vi "findNodesFromPath.vi"(8 "error in (no error)":errorcluster, 10 "searchInElement":string="/device_settings/analog_output name=\"Ao32\"", 11 "xmlNode in":refnum<class "xmlNode.lvclass">) -> (0 "error out":errorcluster, 1 "rest of xml":string, 2 "xmlNode":refnum<class "xmlNode.lvclass">, 3 "xmlNode out":refnum<class "xmlNode.lvclass">, 5 "xml before":string)   [LabVIEW 2011, in "Tools.lvlib" / "xml.lvlib" / "xmlNode.lvclass"]
uses:
  xmlNode.lvclass
  XmlParser.lvclass
panel:
  out "xml":string
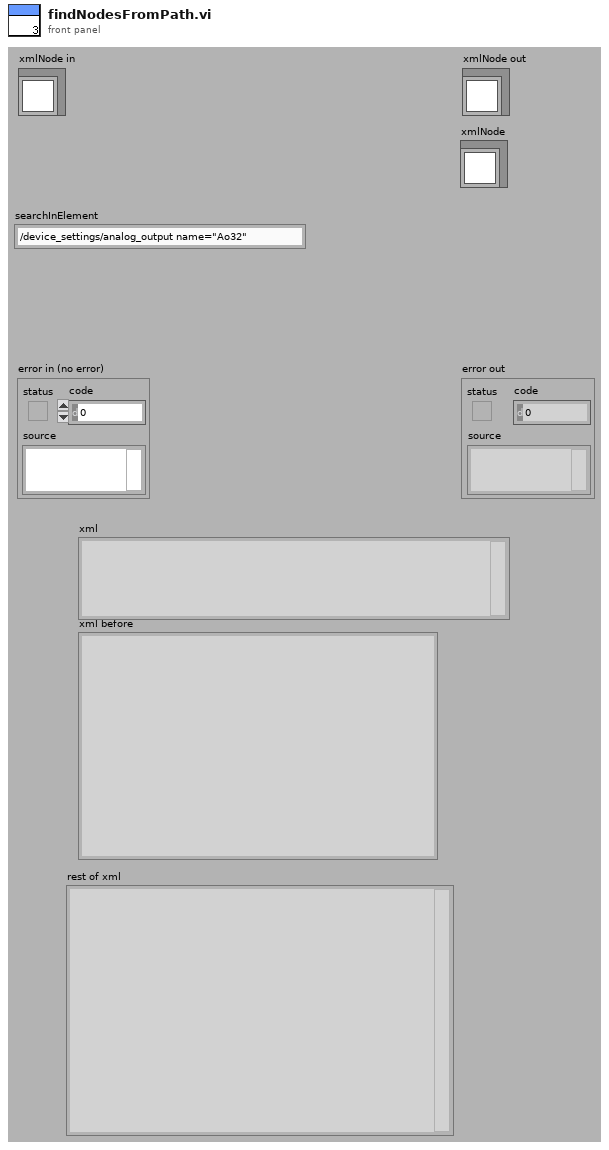
[diagram p1: front panel]
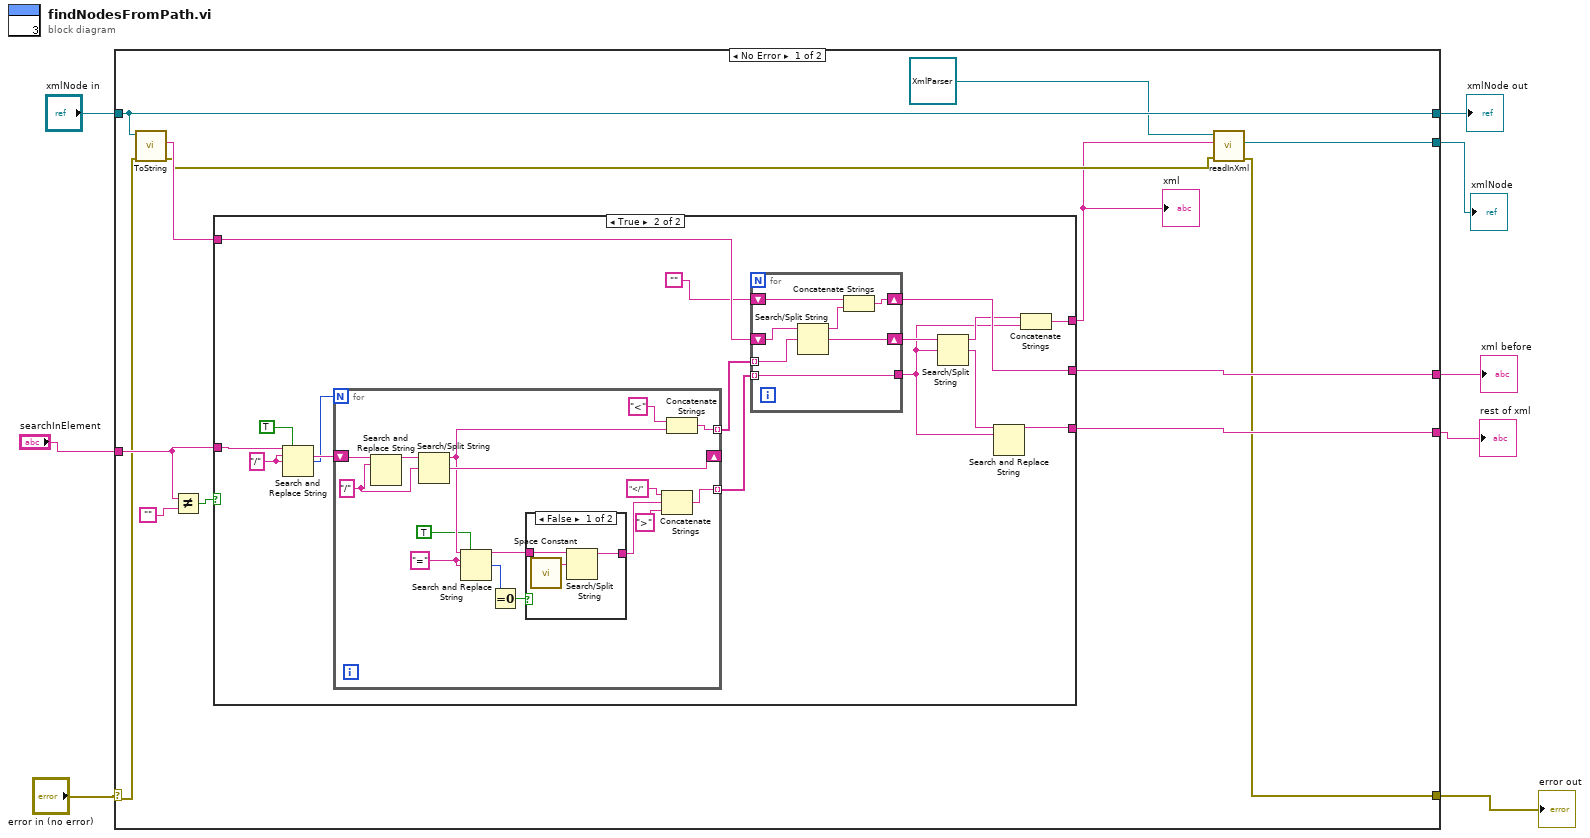
[diagram p0: block diagram]
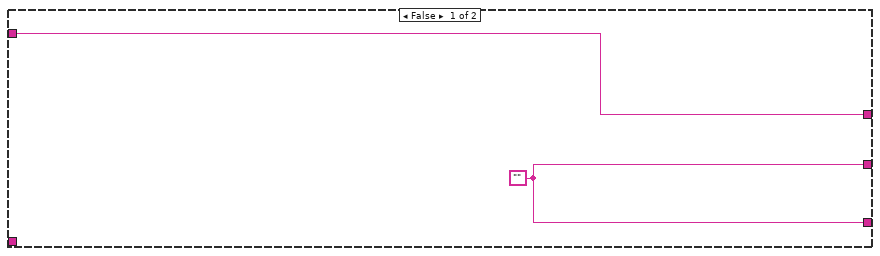
[diagram p2: hidden frame]
diagram:
  n1 = case shown="No Error" "error in (no error)" {
    selector: "error in (no error)" -> [w12 w68]
    tunnel: [w10 w68] -> w7
    tunnel: [w18 w67] -> w5
    tunnel: "xmlNode in" -> [w18 w67]
    tunnel: "searchInElement" -> [w19 _]
    tunnel: [w16 _] -> w2
    tunnel: [w15 _] -> w1
    tunnel: [w11 _] -> w3
    frame No Error {
      n2 = call-dynamic "ToString.vi"("error in (no error)"=w12, "xmlNode in"=w18) -> ("error out"=w13:errorcluster, "xml"=w17:string)  [unwired: 7 in, 1 out]
      n3 = Not Equal?(x=w19, y="") -> (x != y?=w20:bool)
      n4 = case shown="True" w20 {
        tunnel: [w22 w34] -> w9
        tunnel: w19 -> [_ w35]
        tunnel: [w23 w24] -> w15
        tunnel: [w23 w30] -> w16
        tunnel: w17 -> [w22 w32]
        frame False {
          w23 = ""
        }
        frame True {
          w37 = "/"
          n5 = Search and Replace String(replace all?=TRUE, input string=w35, search string=w37, replace string=w37) -> (result string=w39:string, number of replacements=w38:i32)  [unwired: 4 in, 2 out]
          n6 = for {
            N: w38 -> [_]
            tunnel: [w56] -> w33 mode=indexing
            tunnel: [w55] -> w27 mode=indexing
            shift-right: [w54] -> _
            shift-left: w39 -> [w62]
            w52 = "="
            w61 = "/"
            n7 = Search and Replace String(input string=w62, search string=w61) -> (result string=w60:string)  [unwired: 6 in, 3 out]
            n8 = Search/Split String(string=w60, search string/char (-)=w61) -> (substring before match=w53:string, match + rest of string=w54:string)  [unwired: 1 in, 1 out]
            n9 = Search and Replace String(replace all?=TRUE, input string=w53, search string=w52, replace string=w52) -> (result string=w49:string, number of replacements=w51:i32)  [unwired: 4 in, 2 out]
            n10 = Equal To 0?(x=w51) -> (x = 0?=w50:bool)
            n11 = case shown="False" w50 {
              tunnel: w49 -> [w65 w66]
              tunnel: [w63 w66] -> w48
              frame False {
                n12 = call <vilib>:"Space Constant.vi"() -> ("String"=w64:string)
                n13 = Search/Split String(string=w65, search string/char (-)=w64) -> (substring before match=w63:string)  [unwired: 1 in, 2 out]
              }
              frame True {
              }
            }
            n14 = Concatenate Strings("</", w48, ">") -> (w55:string)
            n15 = Concatenate Strings("<", w53) -> (w56:string)
          }
          n16 = for {
            tunnel: w33 -> [w41] mode=indexing
            shift-right: [w44] -> w30
            shift-left: "" -> [w45]
            shift-right: [w42] -> w29
            shift-left: w32 -> [w46]
            tunnel: [w40] -> w25
            tunnel: w27 -> [w40] mode=indexing
            n17 = Search/Split String(string=w46, search string/char (-)=w41) -> (substring before match=w43:string, match + rest of string=w42:string)  [unwired: 1 in, 1 out]
            n18 = Concatenate Strings(w45, w43) -> (w44:string)
          }
          n19 = Search/Split String(string=w29, search string/char (-)=w25) -> (substring before match=w28:string, match + rest of string=w26:string)  [unwired: 1 in, 1 out]
          n20 = Search and Replace String(input string=w26, search string=w25) -> (result string=w24:string)  [unwired: 6 in, 3 out]
          n21 = Concatenate Strings(w28, w25) -> (w34:string)
        }
      }
      "xml" <- w9
      n22 = call "readInXml.vi"("error in (no error)"=w13, "xmlString"=w9, "XmlParser in"=refnum<class "XmlParser.lvclass"> refnum ("Tools.lvlib:XmlParser.lvclass")) -> ("error out"=w10:errorcluster, "xmlNode"=w11:refnum<class "xmlNode.lvclass">)  [unwired: 6 in, 1 out]
    }
    frame Error {
    }
  }
  "error out" <- w7
  "xmlNode out" <- w5
  "xmlNode" <- w3
  "xml before" <- w2
  "rest of xml" <- w1
